vi "Get dinero.vi"(8 "error in (no error)":errorcluster, 10 "Dinero":dbl, 11 "User Interface in":refnum<class "User Interface.lvclass">) -> (0 "error out":errorcluster, 3 "User Interface out":refnum<class "User Interface.lvclass">)   [LabVIEW 2020, in "User Interface.lvlib" / "User Interface.lvclass"]
uses:
  User Interface.lvclass
  Paquetes Disonibles Messages/Get credit available Msg/Get credit available Msg.lvclass
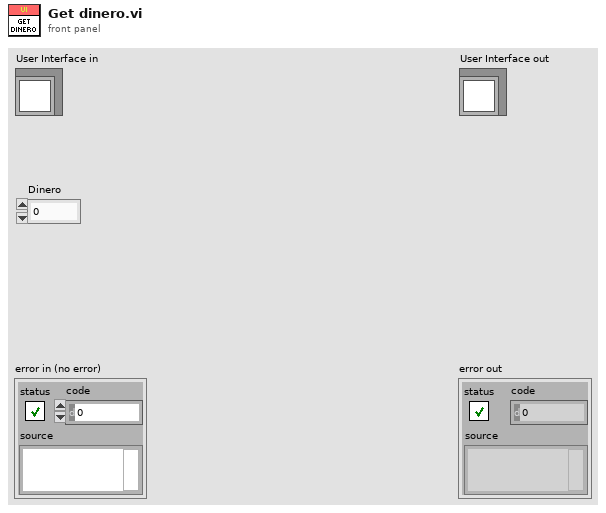
[diagram p1: front panel]
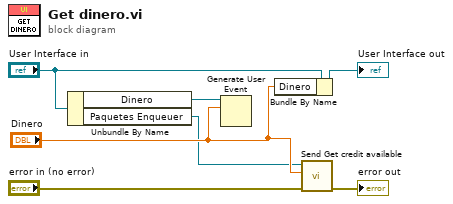
[diagram p0: block diagram]
diagram:
  n1 = Unbundle By Name("User Interface in") -> ("Dinero"=w6:refnum<user-event>, "Paquetes Enqueuer"=w3:refnum<class "Message Enqueuer.lvclass">)
  n2 = Generate User Event(user event=w6, event data cluster="Dinero") -> ()  [unwired: 2 in, 2 out]
  n3 = Bundle By Name(cluster="User Interface in", "Dinero"="Dinero") -> (→"User Interface out":refnum<class "User Interface.lvclass">)
  n4 = call "Send Get credit available.vi"("error in (no error)"="error in (no error)", "Credito Disponible"="Dinero", "Message Enqueuer"=w3) -> ("error out"=→"error out":errorcluster)  [unwired: 7 in, 1 out]
